vi "stage_calibration.vi"() -> ()   [LabVIEW 2014]
uses:
  <vilib>/Utility/file.llb/Read From Spreadsheet File (DBL).vi
panel:
  in  "Sensor type":enum16{"ASAP", "ILEMT"}(ring)=enum."ILEMT"
  in  "Settling time":dbl=1.0
  out "Out OK":bool
  out "In OK":bool
  in  "Run":bool
  in  "Input mode":enum16{"Absolute axis", "Relative axis", "Pose"}(ring)=enum."Pose"
  out "Points done":i32
  out "# Points":i32
  out "Position":dbl[](array[numeric]) format="%#_3p"
  out "State":enum16{"Initialize", "Move", "Log", "Done"}(ring)
  in  "Axis names":string[](array[string])=["X", "Y", "Z", "Rx", "Ry", "Rz"]
  in  "Axis enable":bool[](array[boolean])=[TRUE, TRUE, TRUE, FALSE, FALSE, TRUE]
  in  "stop":bool
  in  "Point time":dbl=1.0
  out "ASAP status":cluster{"Valid position":bool, "Message":string}
  in  "Output file":path=path "D:/Micron/magnetic/Matlab/calibrate_out.dat"
  in  "Input points file":path=path "D:/Micron/magnetic/Matlab/calibrate_in.dat"
  # "Calibration motion controller"
  # "Point"
  # "of"
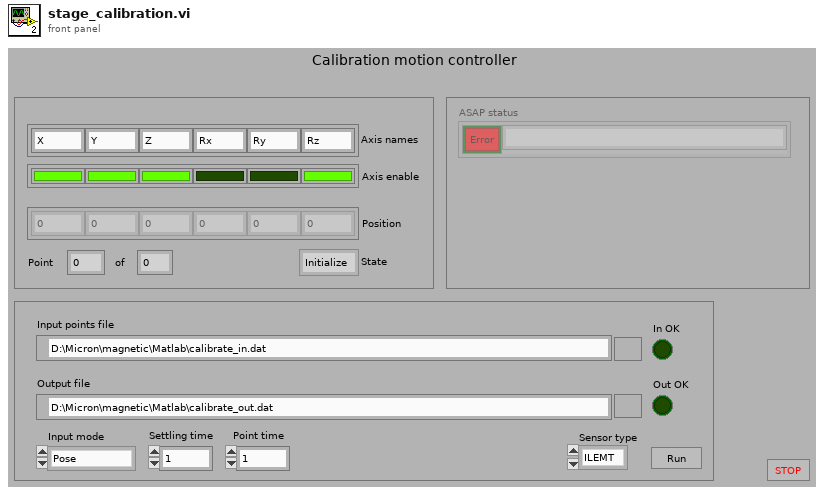
[diagram p1: front panel]
types:
  T1 = enum16{"open", "replace", "create", "open or create", "replace or create", "replace or create with confirmation"}
  T2 = typedef "motion_status.ctl" = cluster{"Axis names":string[], "Axis positions":dbl[], "Pose":dbl[], "Timestamp":u32, "Ready":bool, "Stopped":bool}
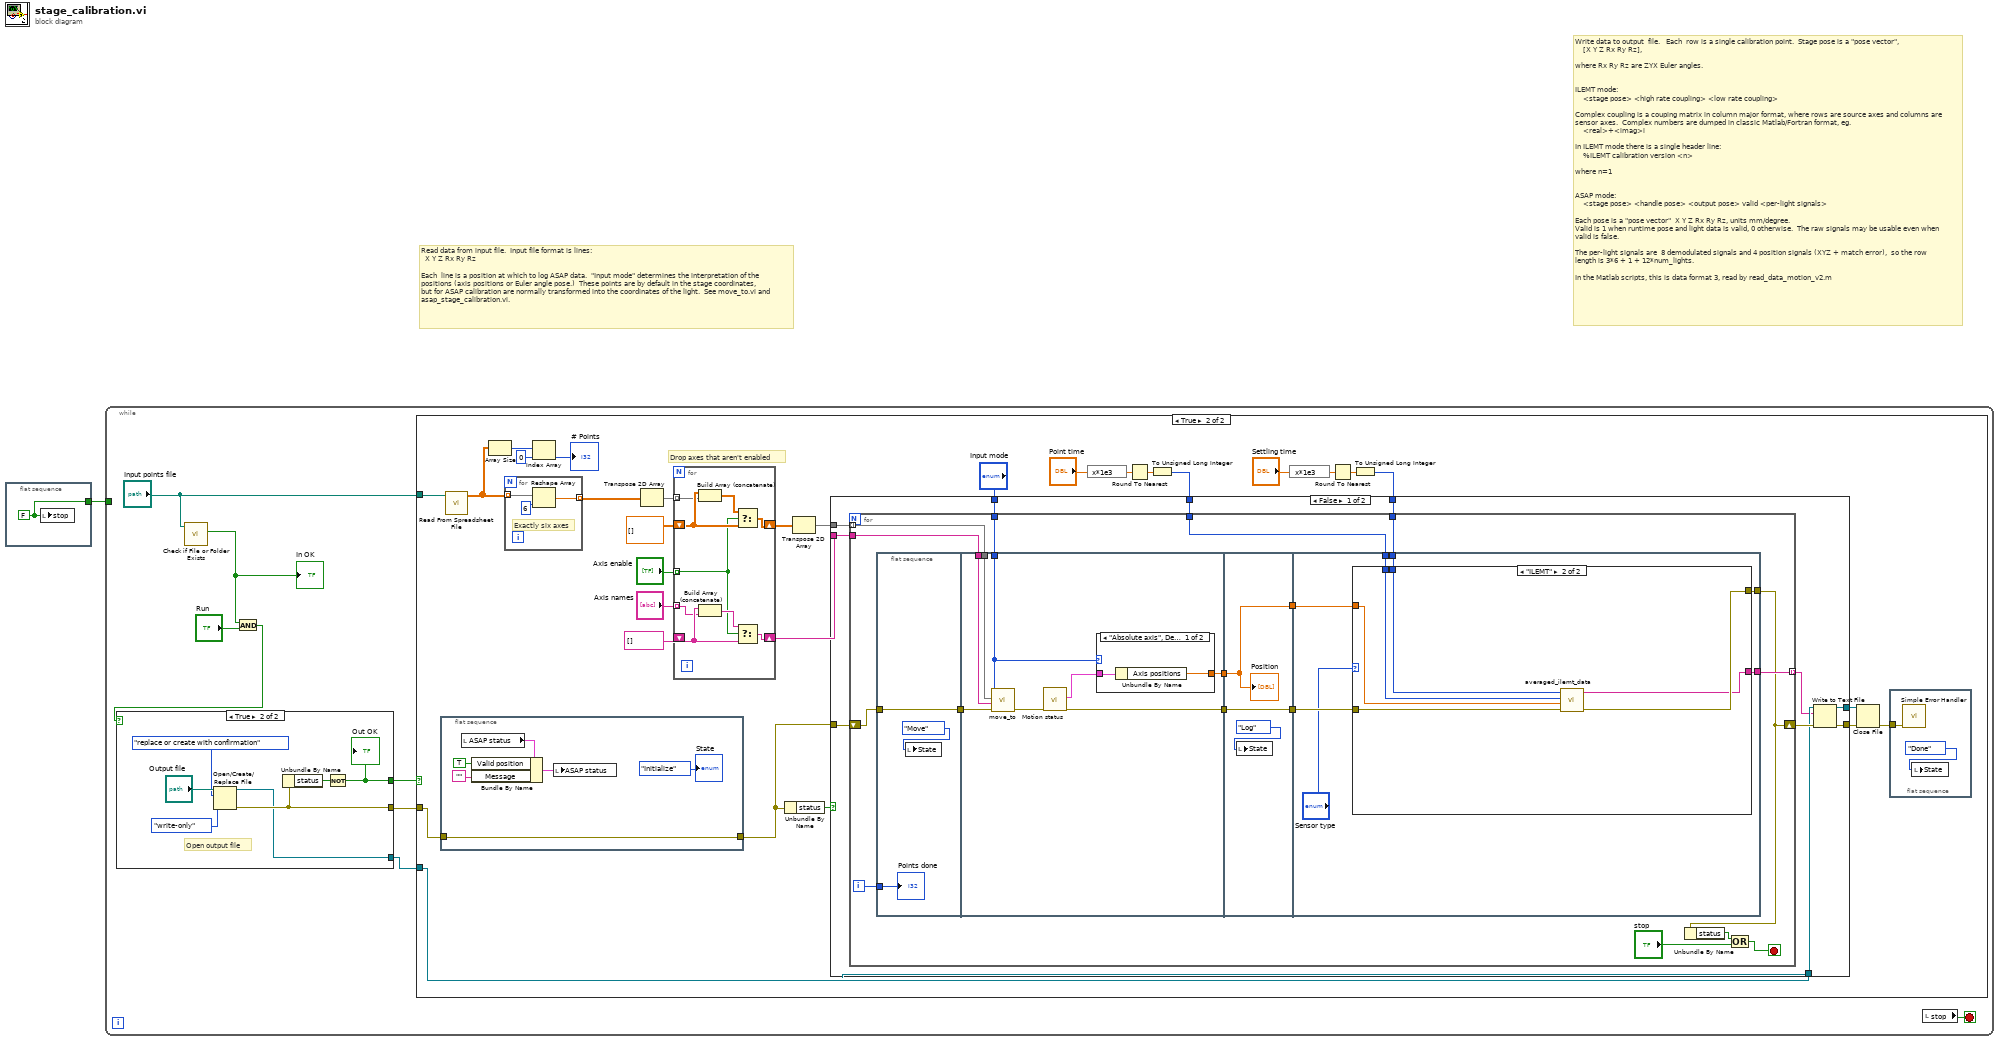
[diagram p0: block diagram]
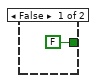
[diagram p2: hidden frame]
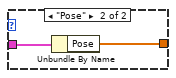
[diagram p4: hidden frame]
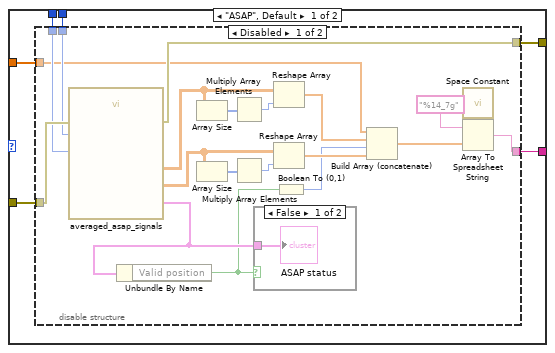
[diagram p5: hidden frame]
diagram:
  # "Write data to output  file.   Each  row is a single calibration point.  Stage pose is a \"pose vector\",\n    [X Y Z Rx Ry Rz],\n\nwhere Rx Ry Rz are ZYX Euler angles.\n\n\nILEMT mode:\n    <stage pose> <high rate coupling> <low rate coupling>\n\nComplex coupling is a couping matrix in column major format, where rows are source axes and columns are sensor axes.  Complex numbers are dumped in classic Matlab/Fortran format, eg. \n    <real>+<imag>i\n\nIn ILEMT mode there is a single header line:\n    %ILEMT calibration version <n>\n\nwhere n=1\n\n\nASAP mode:\n    <stage pose> <handle pose> <output pose> valid <per-light signals>\n\nEach pose is a \"pose vector\"  X Y Z Rx Ry Rz, units mm/degree.\nValid is 1 when runtime pose and light data is valid, 0 otherwise.  The raw signals may be usable even when valid is false.\n\nThe per-light signals are  8 demodulated signals and 4 position signals (XYZ + match error),  so the row length is 3*6 + 1 + 12*num_lights.\n\nIn the Matlab scripts, this is data format 3, read by read_data_motion_v2.m"
  # "Read data from input file.  Input file format is lines:\n  X Y Z Rx Ry Rz\n\nEach  line is a position at which to log ASAP data.  \"Input mode\" determines the interpretation of the positions (axis positions or Euler angle pose.)  These points are by default in the stage coordinates, but for ASAP calibration are normally transformed into the coordinates of the light.  See move_to.vi and asap_stage_calibration.vi."
  n1 = flat-sequence {
    tunnel: [w2] -> w1
    frame #0 {
      w2 = FALSE ("stop")
      n2 = local write "stop"(w2) -> ()
    }
  }
  n3 = while {
    tunnel: w1 -> [_]
    stop <- w7 stop-if-true
    n4 = call <vilib>:"Check if File or Folder Exists.vi"("path"="Input points file") -> ("file or folder exists?"=w3:bool)  [unwired: 8 in, 2 out]
    "In OK" <- w3
    n5 = And(x=w3, y="Run") -> (x .and. y?=w5:bool)
    n6 = case shown="True" w5 {
      tunnel: [_ w18] -> w9
      tunnel: [_ w17] -> w8
      tunnel: [FALSE w12] -> w4
      frame False {
      }
      frame True {
        # "Open output file"
        n7 = Open/Create/Replace File(file path (use dialog)="Output file", operation (0:open)=T1."replace or create with confirmation", access (0:read/write)=enum16{"read/write", "read-only", "write-only"}."write-only") -> (refnum out=w17:refnum<file>, error out=w18:errorcluster)  [unwired: 3 in, 1 out]
        n8 = Unbundle By Name(w18) -> ("status"=w16:bool)
        n9 = Not(x=w16) -> (.not. x?=w12:bool)
        "Out OK" <- w12
      }
    }
    n10 = case shown="True" w4 {
      tunnel: "Input points file" -> [_ w47]
      tunnel: w9 -> [_ w31]
      tunnel: w8 -> [_ w33]
      frame False {
      }
      frame True {
        # "Drop axes that aren't enabled"
        n11 = flat-sequence {
          tunnel: w31 -> [w57]
          tunnel: [w57] -> w30
          frame #0 {
            n12 = local read "ASAP status"() -> (w53:cluster{"Valid position":bool, "Message":string})
            n13 = Bundle By Name(cluster=w53, "Valid position"=TRUE, "Message"="") -> (w55:cluster{"Valid position":bool, "Message":string})
            n14 = local write "ASAP status"(w55) -> ()
            "State" <- enum16{"Initialize", "Move", "Log", "Done"}."Initialize" ("State")
          }
        }
        n15 = call-poly <vilib>:"Read From Spreadsheet File.vi"("file path (dialog if empty)"=w47) -> ("all rows"=w29:dbl[][])  [unwired: 6 in, 4 out]
        n16 = Array Size(array=w29) -> (size(s)=w36:i32[])
        n17 = for {
          tunnel: w29 -> [w51] mode=indexing
          tunnel: [w49] -> w27 mode=indexing
          # "Exactly six axes"
          n18 = Reshape Array(w51, 6 ("dimension size")) -> (w49:dbl[])
        }
        n19 = Index Array(array=w36, index=0) -> (element=→"# Points":i32)
        n20 = Transpose 2D Array(2D array=w27) -> (transposed array=w41:dbl[][])
        n21 = for {
          shift-right: [w65] -> w35
          shift-left: dbl[][] [] ("all rows") -> [w68]
          tunnel: "Axis enable" -> [w60] mode=indexing
          tunnel: w41 -> [w67] mode=indexing
          shift-right: [w61] -> w38
          shift-left: string[] [] ("Axis names") -> [w63]
          tunnel: "Axis names" -> [w62] mode=indexing
          n22 = Build Array (concatenate)(w68, w67) -> (w66:dbl[][])
          n23 = Build Array (concatenate)(w63, w62) -> (w64:string[])
          n24 = Select(t=w66, s=w60, f=w68) -> (s? t:f=w65:dbl[][])
          n25 = Select(t=w64, s=w60, f=w63) -> (s? t:f=w61:string[])
        }
        n26 = Unbundle By Name(w30) -> ("status"=w48:bool)
        n27 = Transpose 2D Array(2D array=w35) -> (transposed array=w34:dbl[][])
        n28 = expression code="x*1e3"("Point time") -> (w25:dbl)
        n29 = Round To Nearest(number=w25) -> (nearest integer value=w24:dbl)
        n30 = To Unsigned Long Integer(number=w24) -> (unsigned 32bit integer=w23:u32)
        n31 = expression code="x*1e3"("Settling time") -> (w21:dbl)
        n32 = Round To Nearest(number=w21) -> (nearest integer value=w22:dbl)
        n33 = To Unsigned Long Integer(number=w22) -> (unsigned 32bit integer=w19:u32)
        n34 = case shown="False" w48 {
          tunnel: w30 -> [w75 w155]
          tunnel: w33 -> [w74 w156]
          tunnel: w34 -> [w79 _]
          tunnel: [w78 w156] -> w46
          tunnel: [w76 w155] -> w45
          tunnel: w38 -> [w73 _]
          tunnel: "Input mode" -> [w72 _]
          tunnel: w23 -> [w71 _]
          tunnel: w19 -> [w70 _]
          frame False {
            n35 = for {
              tunnel: w79 -> [w88] mode=indexing
              tunnel: [w96] -> w69 mode=indexing
              shift-right: [w87] -> w77
              shift-left: w75 -> [w95]
              tunnel: w73 -> [w90]
              tunnel: w72 -> [w85]
              tunnel: w71 -> [w83]
              tunnel: w70 -> [w82]
              i -> [w86]
              stop <- w84 stop-if-true
              n36 = flat-sequence {
                tunnel: w95 -> [w99]
                tunnel: [w99] -> w92
                tunnel: w86 -> [w97]
                tunnel: w92 -> [w107]
                tunnel: [w103] -> w91
                tunnel: w90 -> [w106]
                tunnel: w88 -> [w105]
                tunnel: w85 -> [w102]
                tunnel: [w100] -> w81
                tunnel: w91 -> [w114]
                tunnel: [w114] -> w89
                tunnel: w81 -> [w112]
                tunnel: [w112] -> w80
                tunnel: [w120] -> w96
                tunnel: w89 -> [w119]
                tunnel: [w121] -> w87
                tunnel: w83 -> [w118]
                tunnel: w82 -> [w117]
                tunnel: w80 -> [w116]
                frame #0 {
                  n37 = local write "State"(enum16{"Initialize", "Move", "Log", "Done"}."Move" ("State")) -> ()
                  "Points done" <- w97
                }
                frame #1 {
                  n38 = call "move_to.vi"("Error in"=w107, "Axis names"=w106, "Axis positions"=w105, "Mode"=w102) -> ("Error out"=w104:errorcluster)  [unwired: 7 in]
                  n39 = call "Motion status.vi"("error in"=w104) -> ("error out"=w103:errorcluster, "Motion status"=w101:T2)  [unwired: 5 in, 4 out]
                  n40 = case shown="\"Absolute axis\", Default" w102 {
                    tunnel: w101 -> [w109 w111]
                    tunnel: [w108 w110] -> w100
                    frame "Absolute axis", Default {
                      n41 = Unbundle By Name(w109) -> ("Axis positions"=w108:dbl[])
                    }
                    frame "Pose" {
                      n42 = Unbundle By Name(w111) -> ("Pose"=w110:dbl[])
                    }
                  }
                }
                frame #2 {
                  n43 = local write "State"(enum16{"Initialize", "Move", "Log", "Done"}."Log" ("State")) -> ()
                  "Position" <- w112
                }
                frame #3 {
                  n44 = case shown="\"ILEMT\"" "Sensor type" {
                    tunnel: [w127 w153] -> w121
                    tunnel: [w122 w152] -> w120
                    tunnel: w119 -> [w126 w154]
                    tunnel: w118 -> [w125 w150]
                    tunnel: w117 -> [w124 w151]
                    tunnel: w116 -> [w123 w149]
                    frame "ASAP", Default {
                      n45 = disable-structure shown="Disabled" {
                        disable-tunnel: [w147 _] -> w127
                        disable-tunnel: w126 -> [w145 _]
                        disable-tunnel: w125 -> [w140 _]
                        disable-tunnel: w124 -> [w139 _]
                        disable-tunnel: w123 -> [w133 _]
                        disable-tunnel: [w128 _] -> w122
                        frame Disabled {
                          n46 = call "averaged_asap_signals.vi"("error in"=w145, "Averaging time (ms)"=w140, "Settling time (ms)"=w139) -> ("error out"=w147:errorcluster, "ASAP diagnostics"=w146:cluster{"Valid position":bool, "Message":string}, "Poses"=w132:sgl[][], "Demodulated averaged"=w142:sgl[][])  [unwired: 5 in]
                          n47 = Unbundle By Name(w146) -> ("Valid position"=w138:bool)
                          n48 = Array Size(array=w132) -> (size(s)=w135:i32[])
                          n49 = Array Size(array=w142) -> (size(s)=w144:i32[])
                          n50 = Multiply Array Elements(1:w135) -> (0:w136:i32)
                          n51 = Multiply Array Elements(1:w144) -> (0:w143:i32)
                          n52 = case shown="False" w138 {
                            tunnel: w146 -> [w148 _]
                            frame False {
                              "ASAP status" <- w148
                            }
                            frame True {
                            }
                          }
                          n53 = Reshape Array(w132, w136) -> (w134:sgl[])
                          n54 = Reshape Array(w142, w143) -> (w141:sgl[])
                          n55 = Boolean To (0,1)(Boolean=w138) -> (0, 1=w137:i16)
                          n56 = Build Array (concatenate)(w133, w134, w137, w141) -> (w129:dbl[])
                          n57 = call <vilib>:"Space Constant.vi"() -> ("String"=w130:string)
                          n58 = Array To Spreadsheet String(delimiter (Tab)=w130, array=w129, 3:"%14_7g" ("format (%.3f)")) -> (spreadsheet string=w128:string)
                        }
                        frame Enabled {
                        }
                      }
                    }
                    frame "ILEMT" {
                      n59 = call "averaged_ilemt_data.vi"("error in"=w154, "Position"=w149, "Point time (ms)"=w150, "Settling time (ms)"=w151) -> ("error out"=w153:errorcluster, "Result string"=w152:string)  [unwired: 6 in]
                    }
                  }
                }
              }
              n60 = Unbundle By Name(w87) -> ("status"=w94:bool)
              n61 = Compound Arithmetic op=OR(w94, "stop") -> (w84:bool)
            }
            n62 = Write to Text File(file (use dialog)=w74, text=w69, error in=w77) -> (refnum out=w78:refnum<file>, error out=w76:errorcluster)  [unwired: 1 in, 1 out]
          }
          frame True {
          }
        }
        n63 = Close File(refnum=w46, error in=w45) -> (error out=w44:errorcluster)  [unwired: 1 out]
        n64 = flat-sequence {
          tunnel: w44 -> [w59]
          frame #0 {
            n65 = call <vilib>:"Simple Error Handler.vi"("error in (no error)"=w59) -> ()  [unwired: 4 in, 5 out]
            n66 = local write "State"(enum16{"Initialize", "Move", "Log", "Done"}."Done" ("State")) -> ()
          }
        }
      }
    }
    n67 = local read "stop"() -> (w7:bool)
  }
